vi "Dateiheader.vi"(1 "Zeilenindex":i32) -> (0 "String":string)   [LabVIEW 2019]
uses:
  Global Variables/Globale Variablen Torque.vi
  Instrument_Setup.vi
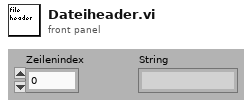
[diagram p1: front panel]
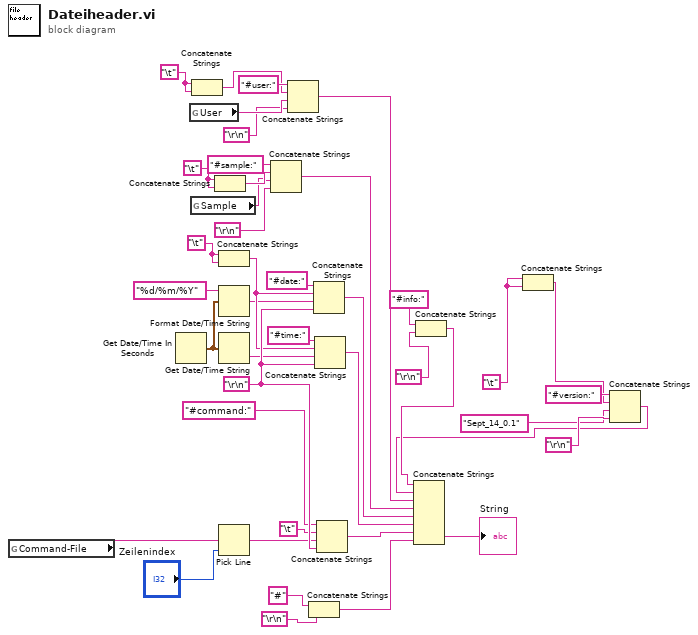
[diagram p0: block diagram]
diagram:
  w5 = "\t"
  w18 = "\t"
  w23 = "\t"
  w38 = "\r\n"
  w30 = "\t"
  n1 = global read "Globale Variablen Torque.vi" "Command-File"() -> (w25:string)
  n2 = Get Date/Time In Seconds() -> (seconds since 1Jan1904=w32:timestamp)
  n3 = global read "Instrument_Setup.vi" "User"() -> (w22:string)
  n4 = global read "Instrument_Setup.vi" "Sample"() -> (w16:string)
  n5 = Concatenate Strings(w23, w23) -> (w20:string)
  n6 = Concatenate Strings(w18, w18) -> (w17:string)
  n7 = Concatenate Strings(w30, w30) -> (w36:string)
  n8 = Format Date/Time String(time format string (%c)="%d/%m/%Y" ("Zeitformatierungs-String (%c)"), seconds (now)=w32) -> (date/time string=w29:string)  [unwired: 1 in]
  n9 = Get Date/Time String(seconds (now)=w32) -> (time string=w33:string)  [unwired: 2 in, 1 out]
  n10 = Pick Line(multi-line string=w25, line index="Zeilenindex") -> (output string=w37:string)  [unwired: 1 in]
  n11 = Concatenate Strings("#sample:" ("String"), w17, w16, "\r\n") -> (w13:string)
  n12 = Concatenate Strings("#user:" ("String"), w20, w22, "\r\n") -> (w14:string)
  n13 = Concatenate Strings("#" ("String"), "\r\n") -> (w10:string)
  n14 = Concatenate Strings("#date:", w36, w29, w38) -> (w39:string)
  n15 = Concatenate Strings("#time:", w36, w33, w38) -> (w40:string)
  n16 = Concatenate Strings("#command:", "\t", w37, w38) -> (w41:string)
  n17 = Concatenate Strings("#info:" ("String"), "\r\n") -> (w7:string)
  n18 = Concatenate Strings(w5, w5) -> (w3:string)
  n19 = Concatenate Strings("#version:" ("String"), w3, "Sept_14_0.1" ("String"), "\r\n") -> (w1:string)
  n20 = Concatenate Strings(w7, w1, w14, w13, w39, w40, w41, w10) -> (→"String":string)
